vi "NameRepository.vi"(8 "error in (no error)":errorcluster, 10 "Names":string[](array[string]), 11 "NameRepository in":refnum<class "NameRepository.lvclass">) -> (0 "error out":errorcluster, 3 "NameRepository out":refnum<class "NameRepository.lvclass">)   [LabVIEW 2016, in "NameRepository.lvclass"]
uses:
  NameRepository.lvclass
  NameRepository.lvclass/NameRepository.ctl
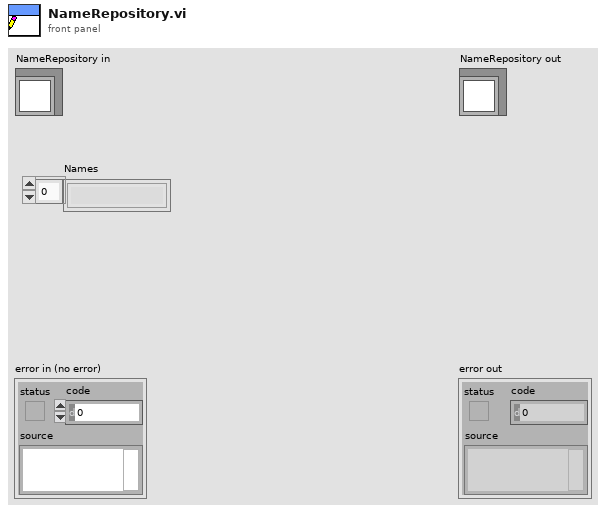
[diagram p1: front panel]
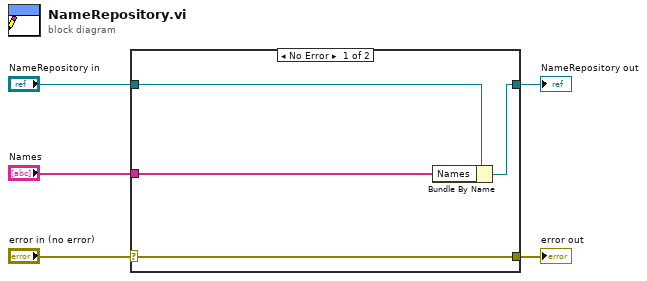
[diagram p0: block diagram]
diagram:
  n1 = case shown="No Error" "error in (no error)" {
    selector: "error in (no error)" -> [w9 w10]
    tunnel: [w9 w10] -> w4
    tunnel: [w7 w11] -> w2
    tunnel: "NameRepository in" -> [w8 w11]
    tunnel: "Names" -> [w6 _]
    frame No Error {
      n2 = Bundle By Name(cluster=w8, "Names"=w6) -> (w7:refnum<class "NameRepository.lvclass">)
    }
    frame Error {
    }
  }
  "error out" <- w4
  "NameRepository out" <- w2
